vi "Simulated Driver (Random Noise).vi"(8 "error in":errorcluster) -> (0 "error out":errorcluster)   [LabVIEW 2017, in "DTACQ - Network Enabled Device Driver.lvlib"]
uses:
  DTACQ - Network Enabled Device Driver.lvlib
  Network Shared Variables/Typedefs/X and Y Variant Arrays--Cluster.ctl
  Network Shared Variables/Shared Variables Library.lvlib
panel:
  out "Frequency (Hz)":dbl format="%#_3p"
  in  "Dataset Length (Samples)":i32=1000 min=2 max=10000
  in  "Idle Time per Cycle (ms)":u32=25
  out "Data Throughput (Bytes/Second)":dbl format="%#_3p"
  in  "stop":bool
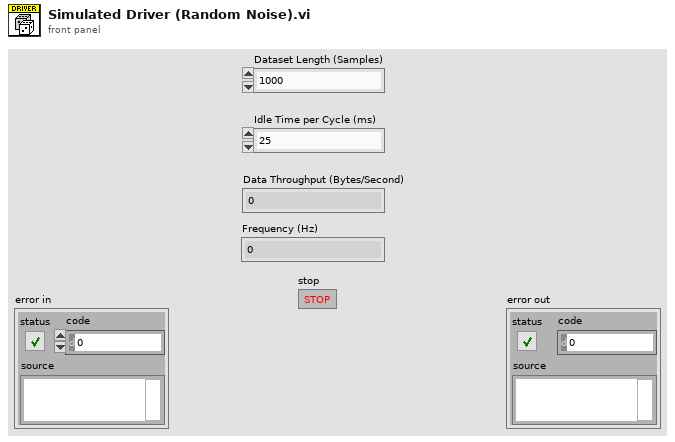
[diagram p1: front panel]
types:
  T1 = typedef "Shared Variables Library.lvlib/X and Y Variant Arrays--Cluster.ctl" = cluster{"X-Data":variant[], "Y-Data":variant[]}
  T2 = cluster{"Read Access":enum8{"Allowed", "Required", "None"}, "Write Access":enum8{"Allowed", "Required", "None"}}
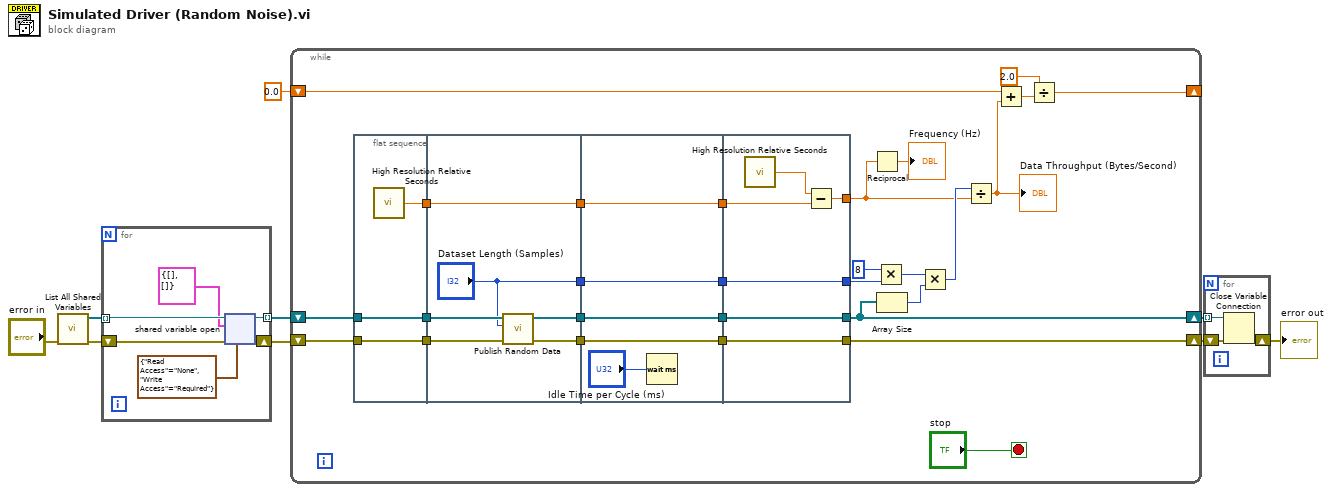
[diagram p0: block diagram]
diagram:
  n1 = call "List All Shared Variables.vi"("error in"="error in") -> ("error out"=w7:errorcluster, "Variable References"=w9:refnum<k21>[])  [unwired: 8 in, 1 out]
  n2 = for {
    tunnel: w9 -> [w15] mode=indexing
    tunnel: [w11] -> w5 mode=indexing
    shift-right: [w10] -> w4
    shift-left: w7 -> [w14]
    n3 = shared-variable-open(w15, w14, T1 {"X-Data"=[], "Y-Data"=[]} ("Data Cluster"), T2 {"Read Access"=enum."None", "Write Access"=enum."Required"} ("access")) -> (w11:refnum<k21>, w10:errorcluster)
  }
  n4 = while {
    shift-right: [w29] -> w2
    shift-left: w5 -> [w40]
    shift-right: [w42] -> w3
    shift-left: w4 -> [w43]
    shift-right: [w30] -> _
    shift-left: 0.0 -> [w34]
    stop <- "stop" stop-if-true
    n5 = flat-sequence {
      tunnel: w40 -> [w45]
      tunnel: w43 -> [w46]
      tunnel: [w46] -> w39
      tunnel: [w45] -> w38
      tunnel: [w44] -> w37
      tunnel: w39 -> [w52]
      tunnel: w38 -> [w49]
      tunnel: [w51] -> w25
      tunnel: [w50] -> w23
      tunnel: w37 -> [w48]
      tunnel: [w48] -> w21
      tunnel: ["Dataset Length (Samples)"] -> w19
      tunnel: w25 -> [w57]
      tunnel: [w57] -> w24
      tunnel: w23 -> [w56]
      tunnel: [w56] -> w22
      tunnel: w21 -> [w55]
      tunnel: [w55] -> w20
      tunnel: w19 -> [w54]
      tunnel: [w54] -> w18
      tunnel: [w62] -> w29
      tunnel: [w63] -> w42
      tunnel: w24 -> [w63]
      tunnel: w22 -> [w62]
      tunnel: w20 -> [w60]
      tunnel: [w59] -> w17
      tunnel: w18 -> [w58]
      tunnel: [w58] -> w36
      frame #0 {
        n6 = call <vilib>:"High Resolution Relative Seconds.vi"() -> ("relative seconds"=w44:dbl)
      }
      frame #1 {
        n7 = call "Publish Random Data.vi"("error in"=w52, "Dataset Length"="Dataset Length (Samples)", "Variable References In"=w49) -> ("error out"=w51:errorcluster, "Variable References Out"=w50:refnum<k21>[])  [unwired: 7 in]
      }
      frame #2 {
        n8 = Wait (ms)(milliseconds to wait="Idle Time per Cycle (ms)") -> ()  [unwired: 1 out]
      }
      frame #3 {
        n9 = call <vilib>:"High Resolution Relative Seconds.vi"() -> ("relative seconds"=w61:dbl)
        n10 = Subtract(x=w61, y=w60) -> (x-y=w59:dbl)
      }
    }
    n11 = Reciprocal(x=w17) -> (1/x=→"Frequency (Hz)":dbl)
    n12 = Multiply(x=8, y=w36) -> (x*y=w27:i32)
    n13 = Array Size(array=w29) -> (size(s)=w28:i32)
    n14 = Multiply(x=w27, y=w28) -> (x*y=w26:i32)
    n15 = Divide(x=w26, y=w17) -> (x/y=w33:dbl)
    "Data Throughput (Bytes/Second)" <- w33
    n16 = Add(x=w34, y=w33) -> (x+y=w32:dbl)
    n17 = Divide(x=2.0, y=w32) -> (x/y=w30:dbl)
  }
  n18 = for {
    tunnel: w2 -> [w64] mode=indexing
    shift-right: [w66] -> w8
    shift-left: w3 -> [w65]
    n19 = Close Variable Connection(8:w65, 11:w64) -> (0:w66:errorcluster)
  }
  "error out" <- w8
